vi "Mark Query.vi"(8 "error in (no error)":errorcluster, 11 "VISA resource name":refnum<visa-resource-name>) -> (0 "error out":errorcluster, 1 "Mark Number":T1, 2 "Mark Point":T2, 3 "VISA resource name out":refnum<visa-resource-name>, 4 "Source Waveform":string, 5 "State":bool, 7 "Mark Owner":string)   [LabVIEW 2016, in "Tektronix DPO MSO 2000 4000 Series.lvlib"]
doc: "Queries the oscilloscope for mark commands.\n\nNote that unlike the <B>Read Marks</B> VI, this returns details about a single marker point."
uses:
  Tektronix DPO MSO 2000 4000 Series.lvlib
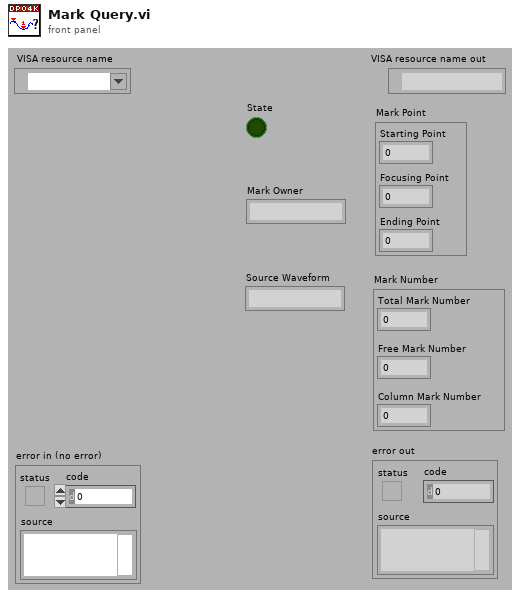
[diagram p1: front panel]
types:
  T1 = cluster{"Free Mark Number":i32, "Total Mark Number":i32, "Column Mark Number":i32}
  T2 = cluster{"Ending Point":dbl, "Focusing Point":dbl, "Starting Point":dbl}
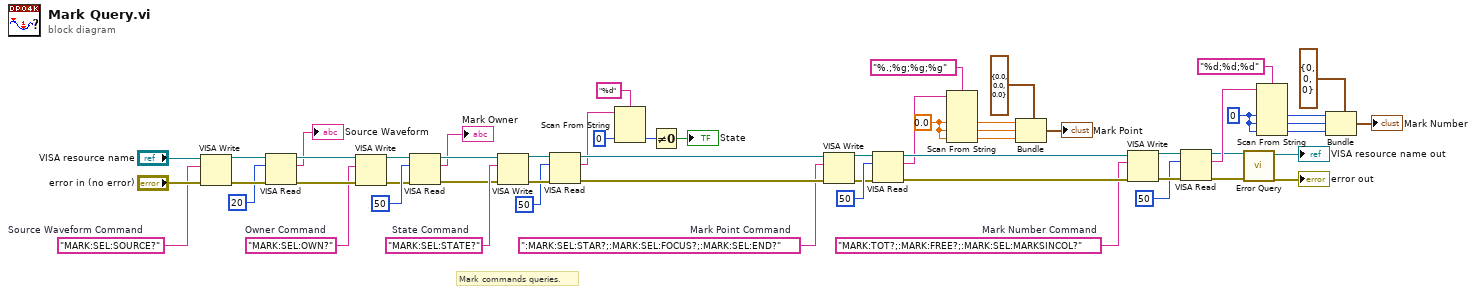
[diagram p0: block diagram]
diagram:
  w3 = 0 ("Column Mark Number")
  w12 = 0.0 ("default value 1")
  w44 = "MARK:SEL:OWN?"  # Owner Command
  w53 = "MARK:SEL:SOURCE?"  # Source Waveform Command
  w40 = "MARK:SEL:STATE?"  # State Command
  w26 = "MARK:TOT?;:MARK:FREE?;:MARK:SEL:MARKSINCOL?"  # Mark Number Command
  w32 = ":MARK:SEL:STAR?;:MARK:SEL:FOCUS?;:MARK:SEL:END?"  # Mark Point Command
  # "Mark commands queries."
  n1 = VISA Write(VISA resource name="VISA resource name", write buffer=w53, error in (no error)="error in (no error)") -> (VISA resource name out=w51:refnum<visa-resource-name>, error out=w52:errorcluster)  [unwired: 1 out]
  n2 = VISA Read(VISA resource name=w51, byte count=u32 20, error in (no error)=w52) -> (VISA resource name out=w46:refnum<visa-resource-name>, read buffer=→"Source Waveform":string, error out=w45:errorcluster)  [unwired: 1 out]
  n3 = VISA Write(VISA resource name=w46, write buffer=w44, error in (no error)=w45) -> (VISA resource name out=w48:refnum<visa-resource-name>, error out=w47:errorcluster)  [unwired: 1 out]
  n4 = VISA Read(VISA resource name=w48, byte count=u32 50, error in (no error)=w47) -> (VISA resource name out=w39:refnum<visa-resource-name>, read buffer=→"Mark Owner":string, error out=w38:errorcluster)  [unwired: 1 out]
  n5 = VISA Write(VISA resource name=w39, write buffer=w40, error in (no error)=w38) -> (VISA resource name out=w42:refnum<visa-resource-name>, error out=w43:errorcluster)  [unwired: 1 out]
  n6 = VISA Read(VISA resource name=w42, byte count=u32 50, error in (no error)=w43) -> (VISA resource name out=w34:refnum<visa-resource-name>, read buffer=w23:string, error out=w33:errorcluster)  [unwired: 1 out]
  n7 = Scan From String(format string="%d", input string=w23, default 1=0 ("default value 1")) -> (output 1=w21:i32)  [unwired: 2 in, 3 out]
  n8 = Not Equal To 0?(x=w21) -> (x != 0?=→"State":bool)
  n9 = VISA Write(VISA resource name=w34, write buffer=w32, error in (no error)=w33) -> (VISA resource name out=w36:refnum<visa-resource-name>, error out=w35:errorcluster)  [unwired: 1 out]
  n10 = VISA Read(VISA resource name=w36, byte count=u32 50, error in (no error)=w35) -> (VISA resource name out=w28:refnum<visa-resource-name>, read buffer=w19:string, error out=w27:errorcluster)  [unwired: 1 out]
  n11 = Scan From String(format string="%.;%g;%g;%g", input string=w19, default 1=w12, default 2=w12, default 3=w12) -> (output 1=w16:dbl, output 2=w15:dbl, output 3=w14:dbl)  [unwired: 2 in, 3 out]
  n12 = Bundle(cluster=T2 {"Ending Point"=0.0, "Focusing Point"=0.0, "Starting Point"=0.0} ("Mark Point"), "Ending Point"=w16, "Focusing Point"=w15, "Starting Point"=w14) -> (→"Mark Point":T2)
  n13 = VISA Write(VISA resource name=w28, write buffer=w26, error in (no error)=w27) -> (VISA resource name out=w30:refnum<visa-resource-name>, error out=w31:errorcluster)  [unwired: 1 out]
  n14 = VISA Read(VISA resource name=w30, byte count=u32 50, error in (no error)=w31) -> (VISA resource name out=w2:refnum<visa-resource-name>, read buffer=w6:string, error out=w1:errorcluster)  [unwired: 1 out]
  n15 = call "Error Query.vi"("error in (no error)"=w1, "VISA resource name"=w2) -> ("error out"=→"error out":errorcluster, "VISA resource name out"=→"VISA resource name out":refnum<visa-resource-name>)  [unwired: 6 in, 2 out]
  n16 = Scan From String(format string="%d;%d;%d", input string=w6, default 1=w3, default 2=w3, default 3=w3) -> (output 1=w8:i32, output 2=w9:i32, output 3=w10:i32)  [unwired: 2 in, 3 out]
  n17 = Bundle(cluster=T1 {"Free Mark Number"=0, "Total Mark Number"=0, "Column Mark Number"=0} ("Mark Number"), "Free Mark Number"=w8, "Total Mark Number"=w9, "Column Mark Number"=w10) -> (→"Mark Number":T1)
